vi "getposition.vi"(1 "COM Port":T1(ring), 2 "Axis":i32=1 min=1 max=6) -> (0 "Position status":dbl format="%.3f")   [LabVIEW 2014]
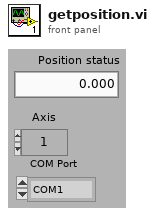
[diagram p1: front panel]
types:
  T1 = enum16{"COM1", "COM2", "COM3", "COM4", "COM5", "COM6", "COM7", "COM8", "COM9"}
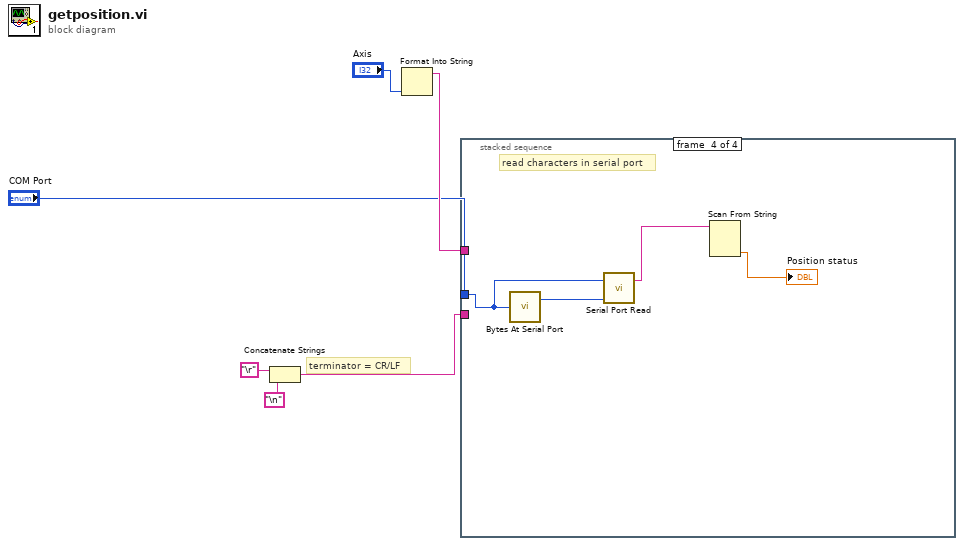
[diagram p0: block diagram]
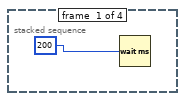
[diagram p2: hidden frame]
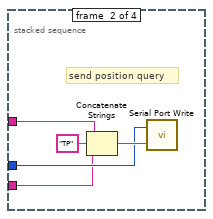
[diagram p3: hidden frame]
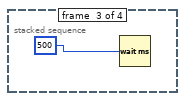
[diagram p4: hidden frame]
diagram:
  # "terminator = CR/LF"
  n1 = Concatenate Strings("\r", "\n") -> (w3:string)
  n2 = Format Into String("Axis") -> (resulting string=w2:string)  [unwired: 3 in, 1 out]
  n3 = stacked-sequence {
    tunnel: w2 -> [_ w10 _ _]
    tunnel: "COM Port" -> [_ w9 _ w14]
    tunnel: w3 -> [_ w8 _ _]
    frame #0 {
      n4 = Wait (ms)(milliseconds to wait=u32 200 ("timeout")) -> ()  [unwired: 1 out]
    }
    frame #1 {
      # "send position query"
      n5 = Concatenate Strings(w10, "TP" ("Substring"), w8) -> (w11:string)
      n6 = call <vilib>:"Serial Port Write.vi"("string to write"=w11, "port number"=w9) -> ()  [unwired: 1 out]
    }
    frame #2 {
      n7 = Wait (ms)(milliseconds to wait=u32 500 ("timeout")) -> ()  [unwired: 1 out]
    }
    frame #3 {
      # "read characters in serial port"
      n8 = call <vilib>:"Bytes At Serial Port.vi"("port number"=w14) -> ("byte count"=w16:u32)  [unwired: 1 out]
      n9 = call <vilib>:"Serial Port Read.vi"("requested byte count"=w16, "port number"=w14) -> ("string read"=w15:string)  [unwired: 1 out]
      n10 = Scan From String(input string=w15) -> (output 1=→"Position status":dbl)  [unwired: 4 in, 3 out]
    }
  }
